vi "New Log.vi"(0 "reference in":refnum<class "Logger.lvclass">, 5 "Logger Data":T1 {"Timestamp Data" format="%<%x %.3X>T"}, 11 "Error In":errorcluster) -> (4 "reference out":refnum<class "Logger.lvclass">, 15 "Error Out":errorcluster)   [LabVIEW 2024, in "Logger.lvclass"]
uses:
  Logger.lvclass
  Logger.lvclass/Logger.ctl
  Support/LoggerData.ctl
panel:
  # "Connector Pane"
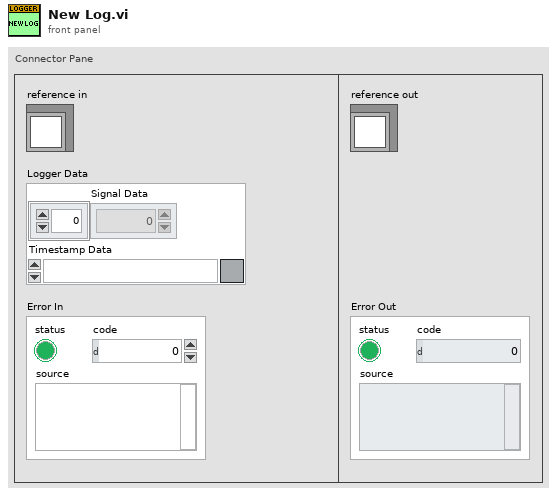
[diagram p1: front panel]
types:
  T1 = typedef "LoggerData.ctl" = cluster{"Signal Data":dbl[], "Timestamp Data":timestamp}
  T2 = typedef "Logger.lvclass/ObjectAttributes.ctl" = cluster{"TDMS File":refnum<k34>, "Channel Names":string[], "Group Name":string}
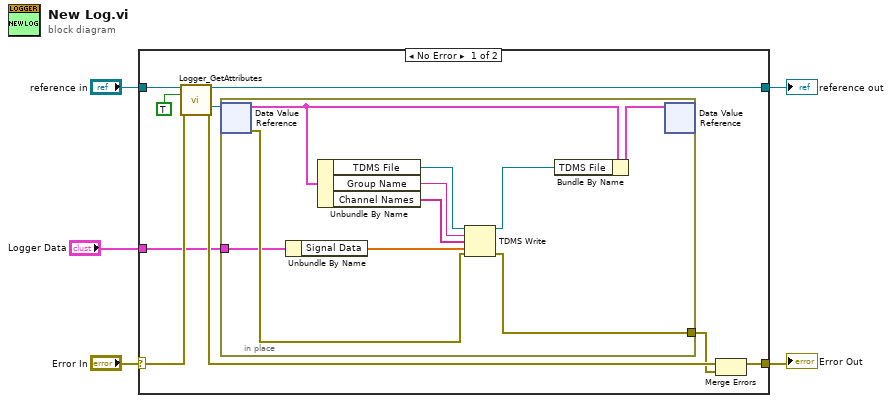
[diagram p0: block diagram]
diagram:
  n1 = case shown="No Error" "Error In" {
    selector: "Error In" -> [w13 w26]
    tunnel: [w11 w26] -> w4
    tunnel: [w12 w25] -> w2
    tunnel: "reference in" -> [w14 w25]
    tunnel: "Logger Data" -> [w6 _]
    frame No Error {
      n2 = call "Logger_GetAttributes.vi"("reference in"=w14, "OnlyGetDvrReference(False)"=TRUE, "Error In"=w13) -> ("reference out"=w12:refnum<class "Logger.lvclass">, "DataRef"=w10:refnum<data-value>, "Error Out"=w9:errorcluster)  [unwired: 9 in, 1 out]
      n3 = in-place {
        in-place-border: [w18] -> w7
        in-place-border: w6 -> [w17]
        n4 = in-place-dvr #1(w10) -> (w23:T2, w19:errorcluster)
        n5 = Unbundle By Name(w17) -> ("Signal Data"=w16:dbl[])
        n6 = Unbundle By Name(w23) -> ("TDMS File"=w22:refnum<k34>, "Group Name"=w21:string, "Channel Names"=w20:string[])
        n7 = TDMS Write(0:w22, 5:w21, 7:w20, 9:w16, 11:w19) -> (4:w15:refnum<k34>, 15:w18:errorcluster)  [unwired: 1 in, 2 out]
        n8 = Bundle By Name(cluster=w23, "TDMS File"=w15) -> (w24:T2)
        n9 = in-place-dvr #1(w24) -> ()  [unwired: 2 out]
      }
      n10 = Merge Errors(w9, w7) -> (w11:errorcluster)
    }
    frame Error {
    }
  }
  "Error Out" <- w4
  "reference out" <- w2
